vi "1-D Gaussian2.vi"(2 "sigma":dbl, 3 "m":dbl, 4 "a":dbl, 5 "x":dbl) -> (0 "y'":dbl[](array[numeric]), 1 "y":dbl)   [LabVIEW 2015]
doc: "1D Gaussian"
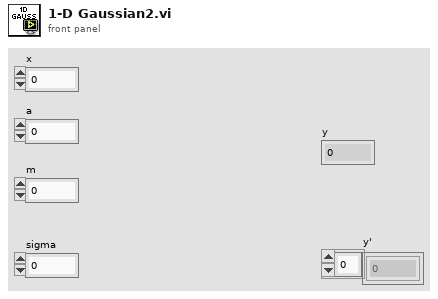
[diagram p1: front panel]
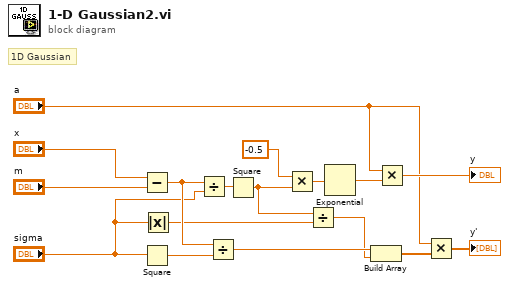
[diagram p0: block diagram]
diagram:
  # "1D Gaussian"
  n1 = Subtract(x="x", y="m") -> (x-y=w12:dbl)
  n2 = Square(x="sigma") -> (x^2=w11:dbl)
  n3 = Absolute Value(x="sigma") -> (abs(x)=w6:dbl)
  n4 = Divide(x=w12, y="sigma") -> (x/y=w17:dbl)
  n5 = Divide(x=w12, y=w11) -> (x/y=w10:dbl)
  n6 = Square(x=w17) -> (x^2=w9:dbl)
  n7 = Multiply(x=-0.5, y=w9) -> (x*y=w15:dbl)
  n8 = Divide(x=w9, y=w6) -> (x/y=w7:dbl)
  n9 = Exponential(1:w15) -> (0:w16:dbl)
  n10 = Build Array(w10, w7) -> (w3:dbl[])
  n11 = Multiply(x="a", y=w16) -> (x*y=→"y":dbl)
  n12 = Multiply(x="a", y=w3) -> (x*y=→"y'":dbl[])
